vi "Close.vi"(8 "error in":errorcluster, 11 "LokiHandler in":refnum<class "LokiHandler.lvclass">) -> (0 "error out":errorcluster, 3 "LokiHandler out":refnum<class "LokiHandler.lvclass">)   [LabVIEW 2017, in "hse-logger.lvlib" / "LokiHandler.lvclass"]
doc: "Tidy up any resources used by the handler. This method should be called when the ``Logger`` gets closed or the handler is removed from the ``Logger``.\n\nThis method is the implementation of the base-class and does nothing."
uses:
  LokiHandler.lvclass
  LokiHandler.lvclass/LokiHandler.ctl
  <vilib>/httpClient/ClientHandle.ctl
  <vilib>/httpClient/LabVIEWHTTPClient.lvlib
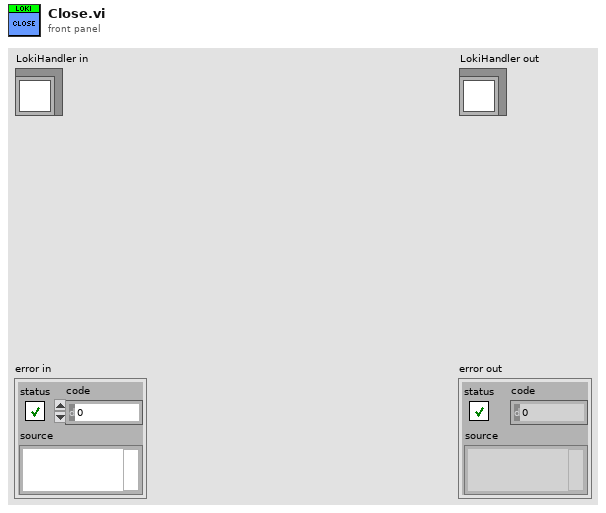
[diagram p1: front panel]
types:
  T1 = typedef "LabVIEWHTTPClient.lvlib/ClientHandle.ctl" = refnum<k1>
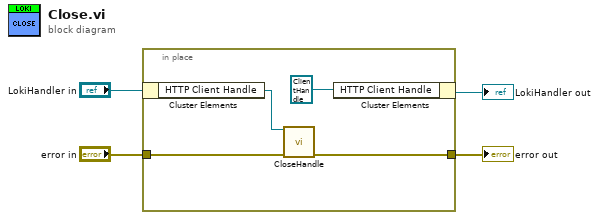
[diagram p0: block diagram]
diagram:
  n1 = in-place {
    in-place-border: "error in" -> [w6]
    in-place-border: [w5] -> w2
    n2 = in-place-cluster #1("LokiHandler in") -> ("HTTP Client Handle"=w7:T1)
    n3 = call <vilib>:"CloseHandle.vi"("client handle"=w7, "error in (no error)"=w6) -> ("error out"=w5:errorcluster)  [unwired: 13 in]
    n4 = in-place-cluster #1("HTTP Client Handle"=T1 refnum) -> (→"LokiHandler out":refnum<class "LokiHandler.lvclass">)
  }
  "error out" <- w2
